vi "DELETE X Minimum Extension.vi"   [LabVIEW 2013]
uses:
  Action.ctl
  Physical Constants FGV Selector.ctl
types:
  T1 = typedef "Physical Constants FGV Selector.ctl" = enum16{"Maximum Output Voltage", "Minimum Output Voltage", "Maximum Input Voltage", "Minimum Input Voltage", "X Piezo Response", "X Piezo Max Extension", "X Piezo Min Extension", "Y Piezo Response", "Y Piezo Max Extension", "Y Piezo Min Extension", "Z Piezo Response", "Z Piezo Max Extension", "Z Piezo Min Extension"}
  T2 = typedef "Action.ctl" = enum16{"GET", "PUT", "DELETE"}
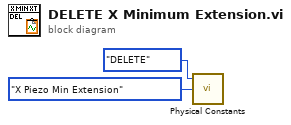
[diagram p0: block diagram]
diagram:
  n1 = call "Physical Constants.vi"("Physical Constants FGV Selector"=Physical_Constants_FGV_Selector."X Piezo Min Extension", "Action"=Action."DELETE") -> ()  [unwired: 1 in, 1 out]
